vi "example_thingspeak”.vi"() -> ()   [LabVIEW 2015]
panel:
  in  "API KEY":string="XXXXXXXXXXX"
  in  "Update Rate (ms)":u32
  in  "Sensor 6 input":dbl
  in  "Sensor 3 input":dbl
  in  "Sensor 4 input":dbl
  in  "Sensor 1 input":dbl
  in  "Sensor 5 input":dbl
  in  "Sensor 2 input":dbl
  # "Send Values for six readings after applying some mathematical operations"
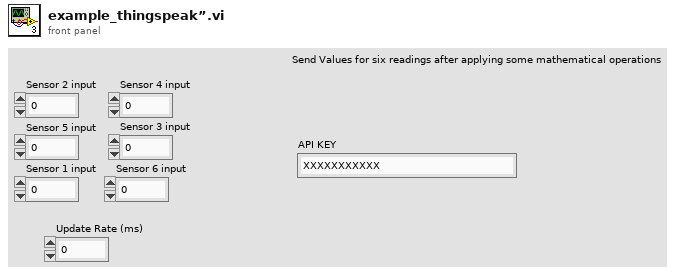
[diagram p1: front panel]
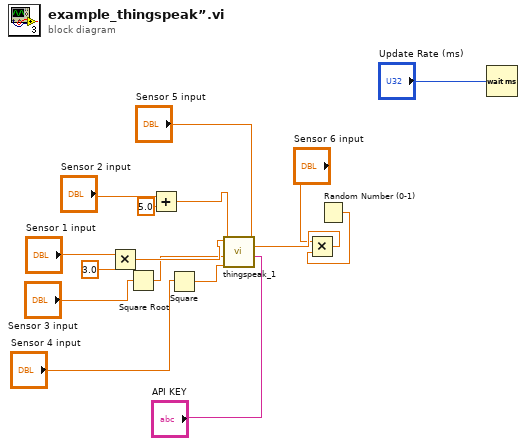
[diagram p0: block diagram]
diagram:
  n1 = Multiply(x="Sensor 1 input", y=3.0) -> (x*y=w14:dbl)
  n2 = Square Root(x="Sensor 3 input") -> (sqrt(x)=w10:dbl)
  n3 = Add(x="Sensor 2 input", y=5.0) -> (x+y=w8:dbl)
  n4 = Square(x="Sensor 4 input") -> (x^2=w12:dbl)
  n5 = Random Number (0-1)() -> (number: 0 to 1=w4:dbl)
  n6 = Multiply(x="Sensor 6 input", y=w4) -> (x*y=w5:dbl)
  n7 = call "thingspeak_1.vi"("Sensor 1 input"=w14, "Sensor 2 input"=w8, "Sensor 3 input"=w10, "Sensor 4 input"=w12, "Sensor 5 input"="Sensor 5 input", "Sensor 6 input"=w5, "API Key"="API KEY") -> ()  [unwired: 4 in]
  n8 = Wait (ms)(milliseconds to wait="Update Rate (ms)") -> ()  [unwired: 1 out]
